vi "Swerve Go To.vi"(0 "Max Speed":dbl, 1 "Target X":dbl, 2 "Target Y":dbl, 3 "Target Angle":dbl) -> (6 "Done":bool)   [LabVIEW 2013]
uses:
  <vilib>/addons/control/pid/pid.llb/PID (DBL).vi
  <vilib>/addons/control/pid/NI_PID_pid.lvlib
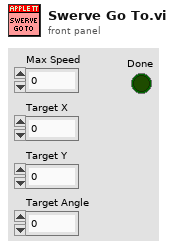
[diagram p1: front panel]
types:
  T1 = enum16{"Prepare to Rotate", "Rotate", "Prepare to Move", "Move"}
  T2 = cluster{"proportional gain (Kc)":dbl, "integral time (Ti, min)":dbl, "derivative time (Td, min)":dbl}
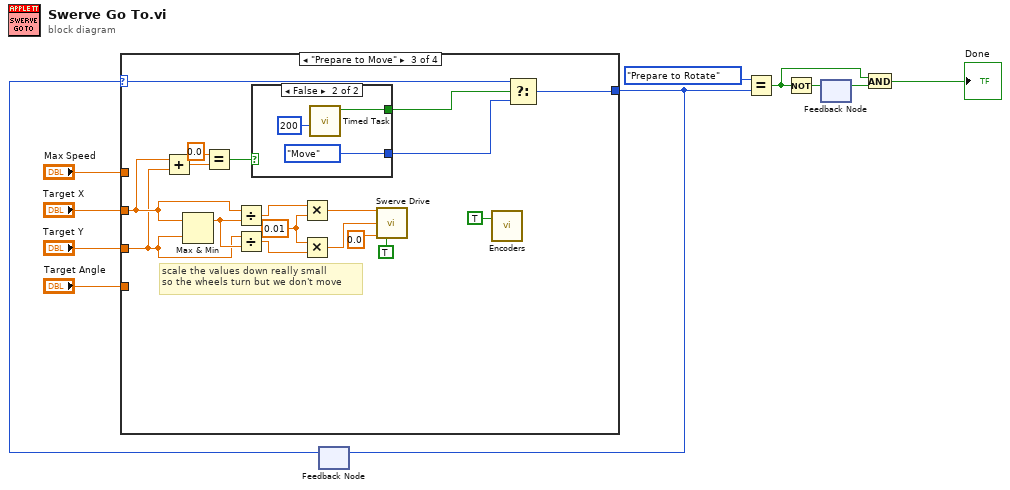
[diagram p0: block diagram]
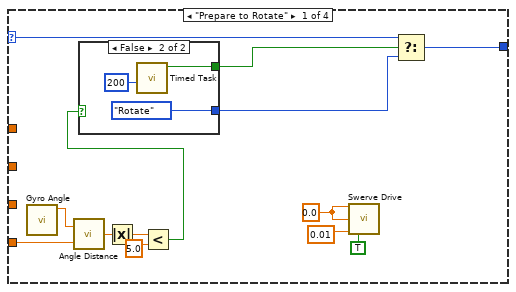
[diagram p2: hidden frame]
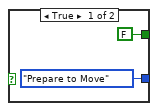
[diagram p3: hidden frame]
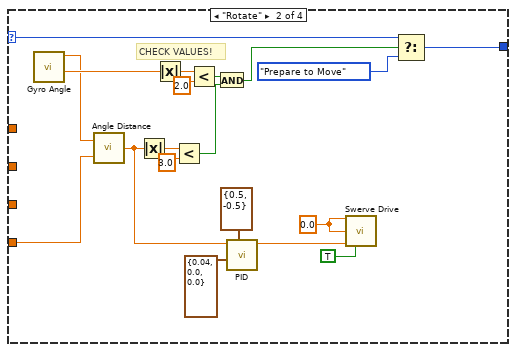
[diagram p4: hidden frame]
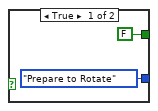
[diagram p5: hidden frame]
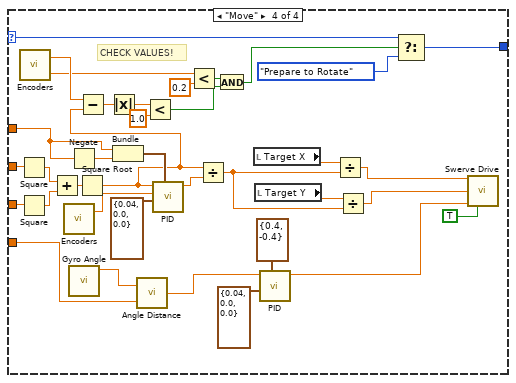
[diagram p6: hidden frame]
diagram:
  n1 = feedback #1() -> (w6:T1)  [unwired: 1 in]
  n2 = case shown="\"Prepare to Move\"" w6 {
    selector: w6 -> [w23 w47 w65 w106]
    tunnel: [w24 w48 w66 w107] -> w4
    tunnel: "Target Angle" -> [w19 w32 _ w76]
    tunnel: "Target X" -> [_ _ w57 w103]
    tunnel: "Target Y" -> [_ _ w56 w102]
    tunnel: "Max Speed" -> [_ _ _ w96]
    frame "Prepare to Rotate" {
      w22 = 0.0
      n3 = call "Gyro Angle.vi"() -> ("Angle"=w20:dbl)  [unwired: 10 in, 1 out]
      n4 = call "Angle Distance.vi"("target angle"=w19, "current angle"=w20) -> ("distance"=w18:dbl)
      n5 = Absolute Value(x=w18) -> (abs(x)=w17:dbl)
      n6 = Less?(x=w17, y=5.0) -> (x < y?=w15:bool)
      n7 = case shown="False" w15 {
        tunnel: [FALSE w28] -> w13
        tunnel: [T1."Prepare to Move" T1."Rotate"] -> w14
        frame True {
        }
        frame False, Default {
          n8 = call "Timed Task.vi"("Time (ms)"=u32 200) -> ("Running"=w28:bool)  [unwired: 10 in]
        }
      }
      n9 = call "Swerve Drive.vi"("X"=w22, "Y"=w22, "Z"=0.01, "Auto Controls"=TRUE) -> ()  [unwired: 12 in]
      n10 = Select(t=w23, s=w13, f=w14) -> (s? t:f=w24:T1)
    }
    frame "Rotate" {
      w45 = 0.0
      # "CHECK VALUES!"
      n11 = call "Gyro Angle.vi"() -> ("Rate"=w35:dbl, "Angle"=w33:dbl)  [unwired: 10 in]
      n12 = call "Angle Distance.vi"("target angle"=w32, "current angle"=w33) -> ("distance"=w31:dbl)
      n13 = Absolute Value(x=w31) -> (abs(x)=w39:dbl)
      n14 = Absolute Value(x=w35) -> (abs(x)=w42:dbl)
      n15 = Less?(x=w39, y=3.0) -> (x < y?=w36:bool)
      n16 = Less?(x=w42, y=2.0) -> (x < y?=w38:bool)
      n17 = And(x=w38, y=w36) -> (x .and. y?=w37:bool)
      n18 = call-poly <vilib>:"PID.vi"("output range"=cluster{"output high":dbl, "output low":dbl} {"output high"=0.5, "output low"=-0.5}, "PID gains"=T2 {"proportional gain (Kc)"=0.04, "integral time (Ti, min)"=0.0, "derivative time (Td, min)"=0.0}, "setpoint"=w31) -> ("output"=w34:dbl)  [unwired: 7 in, 1 out]
      n19 = call "Swerve Drive.vi"("X"=w45, "Y"=w45, "Z"=w34, "Auto Controls"=TRUE) -> ()  [unwired: 12 in]
      n20 = Select(t=w47, s=w37, f=T1."Prepare to Move") -> (s? t:f=w48:T1)
    }
    frame "Prepare to Move" {
      w63 = 0.01 ("y")
      # "scale the values down really small\nso the wheels turn but we don't move"
      n21 = Add(x=w57, y=w56) -> (x+y=w55:dbl)
      n22 = Max & Min(x=w57, y=w56) -> (max(x,y)=w64:dbl)  [unwired: 1 out]
      n23 = Equal?(x=0.0, y=w55) -> (x = y?=w53:bool)
      n24 = Divide(x=w57, y=w64) -> (x/y=w61:dbl)
      n25 = Divide(x=w56, y=w64) -> (x/y=w62:dbl)
      n26 = case shown="False" w53 {
        tunnel: [FALSE w70] -> w51
        tunnel: [T1."Prepare to Rotate" T1."Move"] -> w52
        frame True {
        }
        frame False, Default {
          n27 = call "Timed Task.vi"("Time (ms)"=u32 200) -> ("Running"=w70:bool)  [unwired: 10 in]
        }
      }
      n28 = Multiply(x=w61, y=w63) -> (x*y=w60:dbl)
      n29 = Multiply(x=w63, y=w62) -> (x*y=w59:dbl)
      n30 = call "Swerve Drive.vi"("X"=w60, "Y"=w59, "Z"=0.0, "Auto Controls"=TRUE) -> ()  [unwired: 12 in]
      n31 = call "Encoders.vi"("Reset All"=TRUE) -> ()  [unwired: 1 in, 2 out]
      n32 = Select(t=w65, s=w51, f=w52) -> (s? t:f=w66:T1)
    }
    frame "Move" {
      # "CHECK VALUES!"
      n33 = Square(x=w103) -> (x^2=w101:dbl)
      n34 = Square(x=w102) -> (x^2=w100:dbl)
      n35 = call "Encoders.vi"() -> ("Avg Absolute Rate"=w72:dbl, "Avg Absolute Distance"=w73:dbl)  [unwired: 2 in]
      n36 = Add(x=w101, y=w100) -> (x+y=w99:dbl)
      n37 = call "Encoders.vi"() -> ("Avg Absolute Distance"=w78:dbl)  [unwired: 2 in, 1 out]
      n38 = Negate(x=w96) -> (-x=w97:dbl)
      n39 = call "Gyro Angle.vi"() -> ("Angle"=w77:dbl)  [unwired: 10 in, 1 out]
      n40 = Square Root(x=w99) -> (sqrt(x)=w84:dbl)
      n41 = Subtract(x=w73, y=w84) -> (x-y=w88:dbl)
      n42 = Absolute Value(x=w88) -> (abs(x)=w89:dbl)
      n43 = Bundle("Max Speed"=w96, w97) -> (w98:cluster{"Max Speed":dbl, dbl})  [unwired: 1 in]
      n44 = call "Angle Distance.vi"("target angle"=w76, "current angle"=w77) -> ("distance"=w75:dbl)
      n45 = Less?(x=w89, y=1.0) -> (x < y?=w86:bool)
      n46 = call-poly <vilib>:"PID.vi"("output range"=w98, "PID gains"=T2 {"proportional gain (Kc)"=0.04, "integral time (Ti, min)"=0.0, "derivative time (Td, min)"=0.0}, "process variable"=w78, "setpoint"=w84) -> ("output"=w92:dbl)  [unwired: 6 in, 1 out]
      n47 = Less?(x=w72, y=0.2) -> (x < y?=w87:bool)
      n48 = Divide(x=w84, y=w92) -> (x/y=w93:dbl)
      n49 = And(x=w87, y=w86) -> (x .and. y?=w85:bool)
      n50 = local read "Target X"() -> (w95:dbl)
      n51 = local read "Target Y"() -> (w94:dbl)
      n52 = call-poly <vilib>:"PID.vi"("output range"=cluster{"output high":dbl, "output low":dbl} {"output high"=0.4, "output low"=-0.4}, "PID gains"=T2 {"proportional gain (Kc)"=0.04, "integral time (Ti, min)"=0.0, "derivative time (Td, min)"=0.0}, "setpoint"=w75) -> ("output"=w79:dbl)  [unwired: 7 in, 1 out]
      n53 = Divide(x=w95, y=w93) -> (x/y=w81:dbl)
      n54 = Divide(x=w94, y=w93) -> (x/y=w80:dbl)
      n55 = Select(t=w106, s=w85, f=T1."Prepare to Rotate") -> (s? t:f=w107:T1)
      n56 = call "Swerve Drive.vi"("X"=w81, "Y"=w80, "Z"=w79, "Auto Controls"=TRUE) -> ()  [unwired: 12 in]
    }
  }
  n57 = feedback-in #1(w4) -> ()
  n58 = Equal?(x=T1."Prepare to Rotate", y=w4) -> (x = y?=w1:bool)
  n59 = Not(x=w1) -> (.not. x?=w3:bool)
  n60 = feedback #2() -> (w2:bool)  [unwired: 1 in]
  n61 = feedback-in #2(w3) -> ()
  n62 = And(x=w1, y=w2) -> (x .and. y?=→"Done":bool)
